vi "ITC Read Sensors.vi"() -> (1 "Sensor 2":dbl format="%.2f", 2 "Sensor 1":dbl format="%.2f")   [LabVIEW 2010]
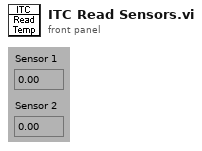
[diagram p1: front panel]
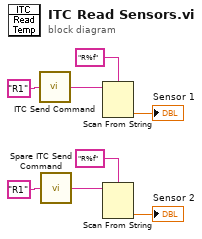
[diagram p0: block diagram]
diagram:
  n1 = call "ITC Send Command.vi"("Command"="R1") -> ("Response"=w6:string)
  n2 = call "Spare ITC Send Command.vi"("Command"="R1") -> ("Response"=w2:string)
  n3 = Scan From String(format string="R%f" ("Format String"), input string=w6) -> (output 1=→"Sensor 1":dbl)  [unwired: 3 in, 3 out]
  n4 = Scan From String(format string="R%f" ("Format String"), input string=w2) -> (output 1=→"Sensor 2":dbl)  [unwired: 3 in, 3 out]
